vi "Unique names.vi"(11 "Names":string[](array[string])) -> (2 "Coma separated":string, 3 "Unique names":string[](array[string]))   [LabVIEW 2015]
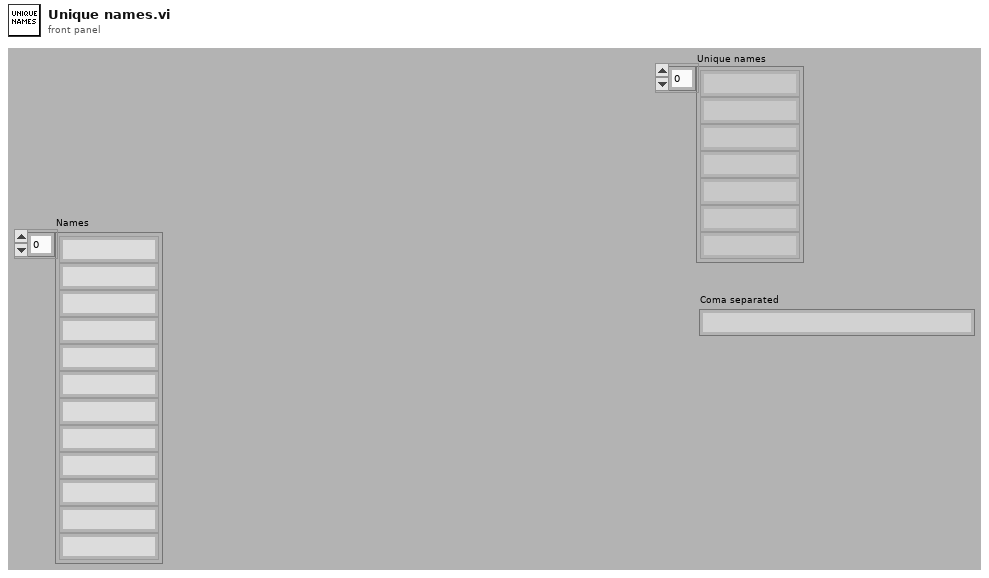
[diagram p1: front panel]
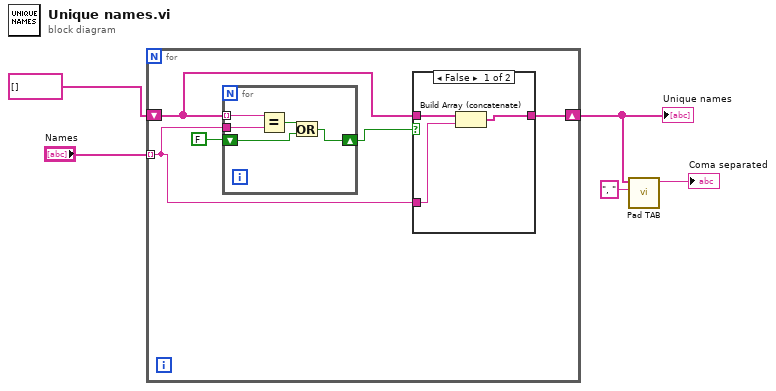
[diagram p0: block diagram]
diagram:
  n1 = for {
    shift-right: [w7] -> w3
    shift-left: string[] [] -> [w8]
    tunnel: "Names" -> [w6] mode=indexing
    n2 = for {
      tunnel: w8 -> [w19] mode=indexing
      tunnel: w6 -> [w18]
      shift-right: [w16] -> w9
      shift-left: FALSE -> [w15]
      n3 = Equal?(x=w19, y=w18) -> (x = y?=w17:bool)
      n4 = Or(x=w17, y=w15) -> (x .or. y?=w16:bool)
    }
    n5 = case shown="False" w9 {
      tunnel: w8 -> [w13 w14]
      tunnel: [w11 w14] -> w7
      tunnel: w6 -> [w12 _]
      frame False {
        n6 = Build Array (concatenate)(w13, w12) -> (w11:string[])
      }
      frame True {
      }
    }
  }
  "Unique names" <- w3
  n7 = call "Pad TAB.vi"("Separator"=", ", "Input String Array"=w3) -> ("Output String"=→"Coma separated":string)  [unwired: 9 in]
